vi "Constants.vi"() -> ()   [LabVIEW 2017, in "NI-SWITCH Shared.lvlib"]
doc: "Use this Global VI to access the GUIDs assigned to the page resources of the Custom Device."
uses:
  NI-SWITCH Shared.lvlib
panel:
  in  "Tab Control":enum32{"GUIDS", "Constants", "Properties"}(tab)
  in  "EndpointConfigGUID":string="c99cfbe4-32a5-4370-896f-695dafdfbaf2"
  in  "NI-SWITCH GUID":string="4ed8d91a-594e-4e06-bfbe-33c7275857dc"
  in  "NI-SWITCH Name":string="NI-SWITCH"
  in  "Compiled.Settings":string="Compiled.Settings"
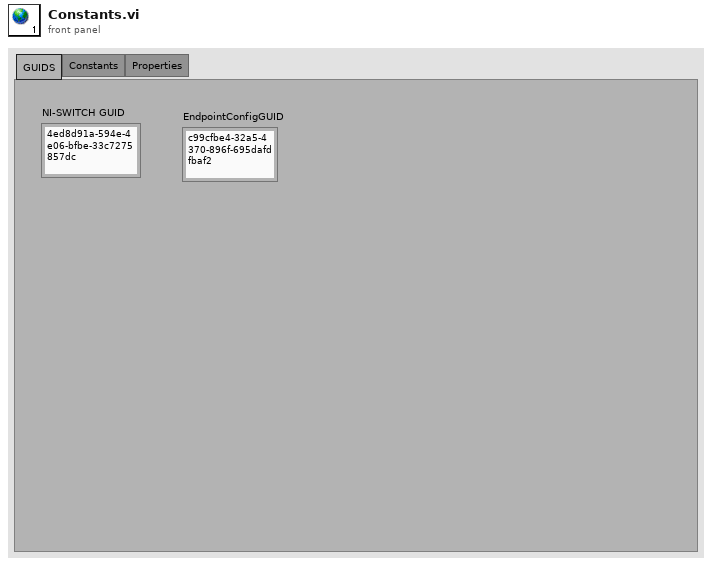
[diagram p1: front panel]
diagram:
